vi "Write PID Controller Values.vi"(7 "Listen Time (s)":sgl=0.1, 8 "error in":errorcluster, 10 "PID":T1={"Ki"=3.65, "Kd"=0.0, "Kp"=0.6}, 11 "Brooks MFC in":refnum<class "Brooks MFC.lvclass">) -> (0 "error out":errorcluster, 2 "PID":T1={"Ki"=3.65, "Kd"=0.0, "Kp"=0.6}, 3 "Brooks MFC out":refnum<class "Brooks MFC.lvclass">)   [LabVIEW 2016, in "Brooks MFC.lvclass"]
uses:
  Brooks MFC.lvclass
  PID.ctl
  Brooks MFC.lvclass/Brooks MFC.ctl
  Instance           3 35Saved   Write PID Controller Values .vi
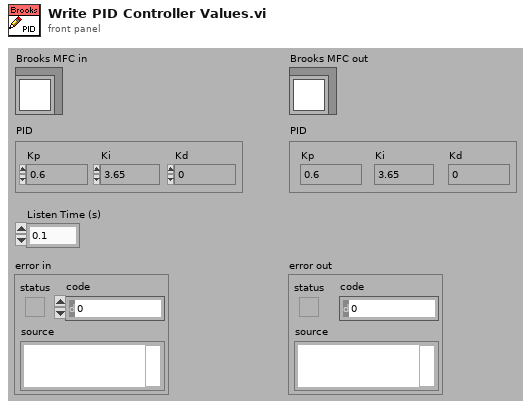
[diagram p1: front panel]
types:
  T1 = typedef "Brooks MFC.lvclass/PID.ctl" = cluster{"Ki":sgl, "Kd":sgl, "Kp":sgl}
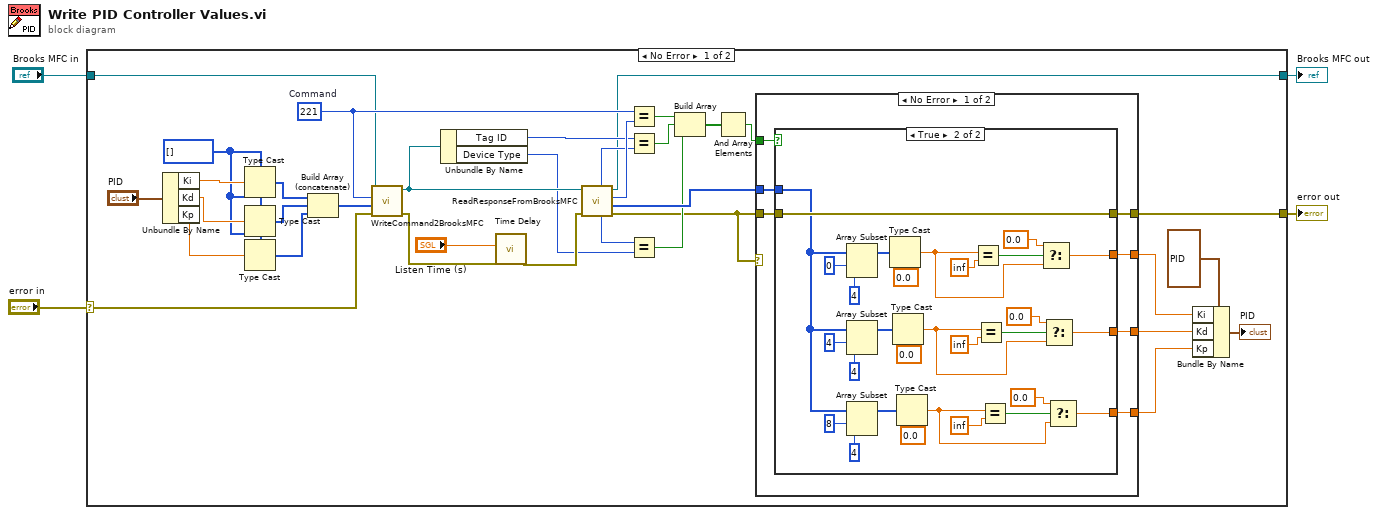
[diagram p0: block diagram]
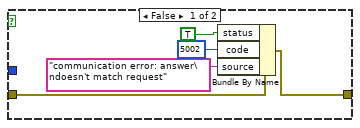
[diagram p2: hidden frame]
diagram:
  n1 = case shown="No Error" "error in" {
    selector: "error in" -> [w9 w82]
    tunnel: "Brooks MFC in" -> [w10 w83]
    tunnel: [w8 w83] -> w1
    tunnel: [w5 w82] -> w2
    frame No Error {
      w27 = u8 221  # Command
      w20 = u8[] [] ("Array")
      n2 = Unbundle By Name("PID") -> ("Ki"=w23:sgl, "Kd"=w22:sgl, "Kp"=w21:sgl)
      n3 = Type Cast(type=w20, x=w23) -> (*(type *) &x=w19:u8[])
      n4 = Type Cast(type=w20, x=w22) -> (*(type *) &x=w18:u8[])
      n5 = Type Cast(type=w20, x=w21) -> (*(type *) &x=w17:u8[])
      n6 = Build Array (concatenate)(w19, w18, w17) -> (w16:u8[])
      n7 = call "WriteCommand2BrooksMFC.vi"("error in"=w9, "Data"=w16, "Command"=w27, "Brooks MFC in"=w10) -> ("error out"=w37:errorcluster, "Brooks MFC out"=w13:refnum<class "Brooks MFC.lvclass">)  [unwired: 5 in, 1 out]
      n8 = Unbundle By Name(w13) -> ("Tag ID"=w12:u32, "Device Type"=w11:u8)
      n9 = call "Time Delay"("error in (no error)"=w37, "Delay Time (s)"="Listen Time (s)") -> ("error out"=w35:errorcluster)  [unwired: 9 in]
      n10 = call "ReadResponseFromBrooksMFC.vi"("error in"=w35, "Brooks MFC in"=w13) -> ("error out"=w15:errorcluster, "Data"=w39:u8[], "Command"=w38:u8, "Brooks MFC out"=w8:refnum<class "Brooks MFC.lvclass">, "device type"=w33:u8, "tag ID"=w34:u32)  [unwired: 4 in]
      n11 = Equal?(x=w27, y=w38) -> (x = y?=w32:bool)
      n12 = Equal?(x=w12, y=w34) -> (x = y?=w31:bool)
      n13 = Equal?(x=w33, y=w11) -> (x = y?=w30:bool)
      n14 = Build Array(w32, w31, w30) -> (w29:bool[])
      n15 = And Array Elements(Boolean array=w29) -> (logical AND=w28:bool)
      n16 = case shown="No Error" w15 {
        tunnel: w15 -> [w46 w81]
        tunnel: w39 -> [w45 _]
        tunnel: [w44 w81] -> w5
        tunnel: w28 -> [w43 _]
        tunnel: [w42 _] -> w26
        tunnel: [w41 _] -> w25
        tunnel: [w40 _] -> w24
        frame No Error {
          n17 = case shown="True" w43 {
            tunnel: w45 -> [_ w54]
            tunnel: w46 -> [w49 w78]
            tunnel: [w48 w78] -> w44
            tunnel: [_ w75] -> w42
            tunnel: [_ w62] -> w41
            tunnel: [_ w52] -> w40
            frame False {
              n18 = Bundle By Name(cluster=w49, "status"=TRUE ("Bundle Element"), "code"=5002 ("Bundle Element"), "source"="communication error: answer\ndoesn't match request") -> (w48:errorcluster)
            }
            frame True {
              n19 = Array Subset(array=w54, index=0 ("Array Index"), length=4 ("Array Length")) -> (w74:u8[])
              n20 = Array Subset(array=w54, index=4 ("Array Index"), length=4 ("Array Length")) -> (w66:u8[])
              n21 = Array Subset(array=w54, index=8 ("Array Index"), length=4 ("Array Length")) -> (w57:u8[])
              n22 = Type Cast(type=sgl 0.0 ("x"), x=w74) -> (*(type *) &x=w72:sgl)
              n23 = Type Cast(type=sgl 0.0 ("x"), x=w66) -> (*(type *) &x=w64:sgl)
              n24 = Type Cast(type=sgl 0.0 ("x"), x=w57) -> (*(type *) &x=w53:sgl)
              n25 = Equal?(x=w72, y=sgl inf ("Single")) -> (x = y?=w77:bool)
              n26 = Equal?(x=w64, y=sgl inf ("Single")) -> (x = y?=w68:bool)
              n27 = Equal?(x=w53, y=sgl inf ("Single")) -> (x = y?=w59:bool)
              n28 = Select(t=sgl 0.0 ("x"), s=w77, f=w72) -> (s? t:f=w75:sgl)
              n29 = Select(t=sgl 0.0 ("x"), s=w68, f=w64) -> (s? t:f=w62:sgl)
              n30 = Select(t=sgl 0.0 ("x"), s=w59, f=w53) -> (s? t:f=w52:sgl)
            }
          }
        }
        frame Error {
        }
      }
      n31 = Bundle By Name(cluster=T1 {"Ki"=3.65, "Kd"=0.0, "Kp"=0.6} ("PID"), "Ki"=w26, "Kd"=w25, "Kp"=w24) -> (→"PID":T1)
    }
    frame Error {
    }
  }
  "error out" <- w2
  "Brooks MFC out" <- w1
